vi "Get Data.vi"(8 "error in":errorcluster, 11 "cCRDS in":refnum<class "cCRDS.lvclass">=refnum) -> (0 "error out":errorcluster, 3 "cCRDS_new out":refnum<class "cCRDS.lvclass">)   [LabVIEW 2015, in "cCRDS.lvclass"]
doc: "Retrieve the data from the given cards. All data is acquired in parallel (from the serial ports and the two analog cards). Set the <B>goodData</B> flag to True and log any errors that will be handled down the line. If there is an error associated with the collection of the data, the <B>goodData</B> flag will be set to false when the logged errors are handled.\nThe ringdown traces recorded in the <B>HF AI</B> task are divided up into a m x n matrix where:\n * m = YAG pulse rate\n * n = YAG duty cycle * HF AI Sampling Rate / YAG Pulse Rate\n\nIn the serial data, the first five elements will be the flow controller data. The first element corresponds to the purge flow with the next as follows: thermodenuded (2), dry (4), med RH (1) and high RH (1). \n\nIn the low frequency data, the first twelve elements correpsond to the T, RH and P in the 4 banks of cells. The T and P measured at the output of the banks is assumed to be constant through the banks. The next two signals are the two humidified inputs and the remaining inputs are reserved for thermistor data."
uses:
  cCRDS.lvclass
  Data/cCRDS Data.lvclass
  Reusable/Instrument/state.ctl
  Data/cCRDS Data.lvclass/cCRDS Data.ctl
  Reusable/CRDS/Data/Cell/calData.ctl
  Reusable/CRDS/Cell/CRDS Cell.lvclass/CRDS Cell.ctl
  Reusable/CRDS/Main/Read Cells.vi
  Data Access/Read LF AI.vi
  Data Access/Read SerialIO.vi
  Reusable/CRDS/Data/Main/Write CellData.vi
  Reusable/CRDS/Main/Write Cells.vi
  Reusable/CRDS/Main/Write goodData.vi
  Reusable/CRDS/Cell/CRDS Cell.lvclass
  Reusable/CRDS/Data/Main/CRDS Data.lvclass
  Devices/Alicat/Session Based/Alicat Device.lvclass
  Reusable/CRDS/Data/Cell/CRDS Cell Data.lvclass
  Reusable/Instrument/Instrument.lvclass
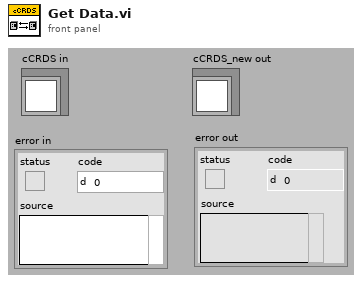
[diagram p1: front panel]
types:
  T1 = typedef "Instrument.lvclass/state.ctl" = enum8{"Configure", "Acquire", "Wait", "Quit", "Handle Error", "NOOP"}
  T2 = typedef "calData.ctl" = cluster{"rhDilFac":sgl, "Q":sgl, "Tmean":sgl, "extDilFac":sgl, "rhCell":sgl, "P":sgl, "T":sgl}
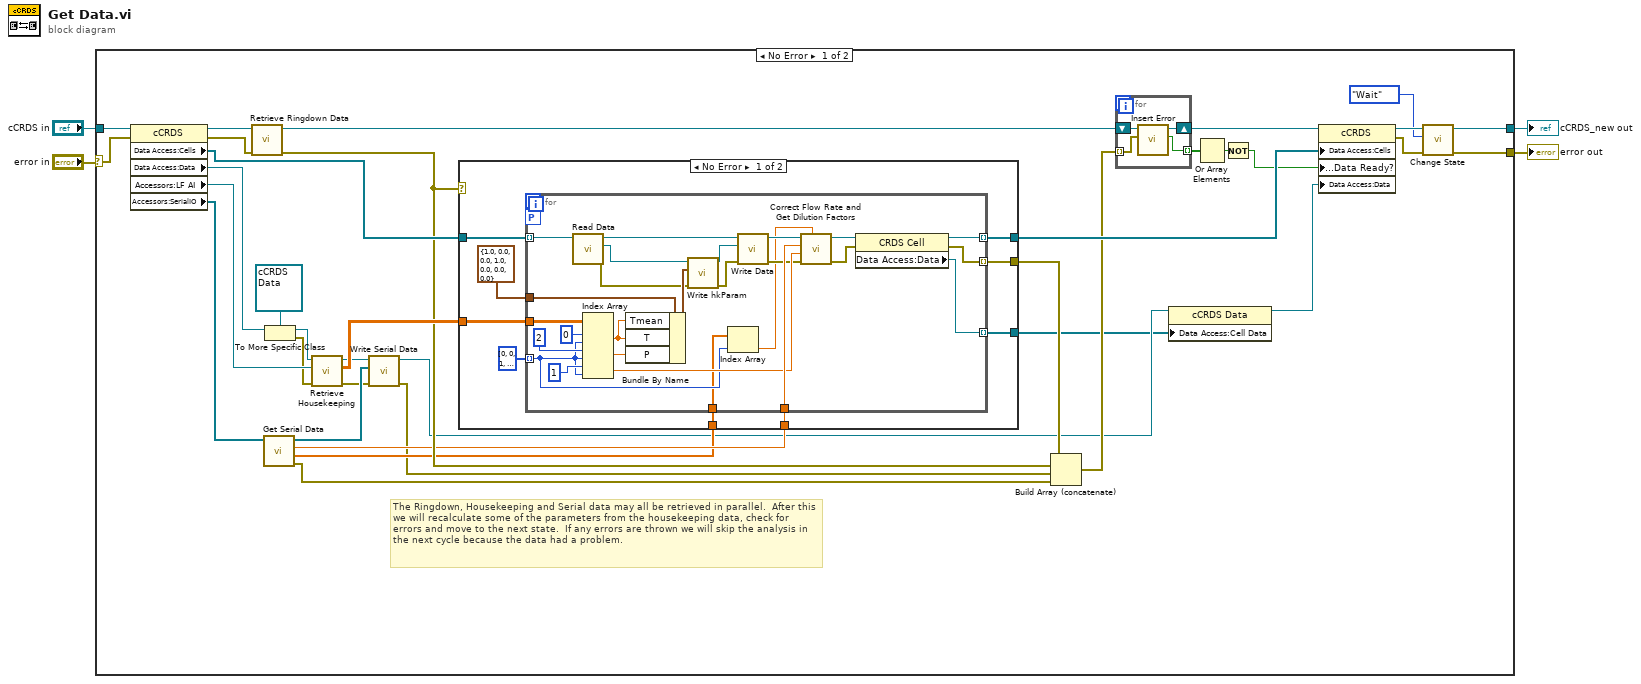
[diagram p0: block diagram]
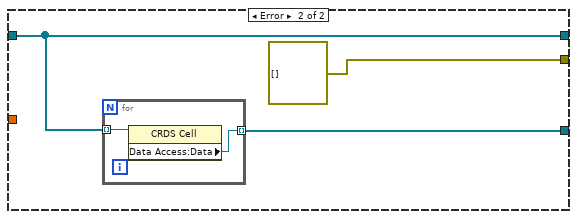
[diagram p2: hidden frame]
diagram:
  n1 = case shown="No Error" "error in" {
    selector: "error in" -> [w39 w86]
    tunnel: [w37 w86] -> w3
    tunnel: "cCRDS in" -> [w40 w85]
    tunnel: [w38 w85] -> w1
    frame No Error {
      # "The Ringdown, Housekeeping and Serial data may all be retrieved in parallel.  After this we will recalculate some of the parameters from the housekeeping data, check for errors and move to the next state.  If any errors are thrown we will skip the analysis in the next cycle because the data had a problem."
      n2 = property class="cCRDS"(reference=w40, error in=w39) -> (reference out=w29:refnum<class "cCRDS.lvclass">, error out=w30:errorcluster, "Data Access:Cells"=w27:refnum<class "CRDS Cell.lvclass">[], "Data Access:Data"=w23:refnum<class "CRDS Data.lvclass">, "Accessors:LF AI"=w26:refnum<k21>, "Accessors:SerialIO"=w12:refnum<class "Alicat Device.lvclass">[])
      n3 = call "Retrieve Ringdown Data.vi"("error in"=w30, "cCRDS in"=w29) -> ("error out"=w20:errorcluster, "cCRDS out"=w28:refnum<class "cCRDS.lvclass">)  [unwired: 8 in]
      n4 = call "Get Serial Data.vi"("SerialIO"=w12) -> ("error out"=w17:errorcluster, "flows"=w18:sgl[], "purge"=w19:sgl, "DataOut"=w10:refnum<class "Data.lvclass">[])  [unwired: 7 in]
      n5 = To More Specific Class(target class=refnum<class "cCRDS Data.lvclass"> refnum ("cCRDS Data"), reference=w23) -> (specific class reference=w25:refnum<class "cCRDS Data.lvclass">, error out=w22:errorcluster)  [unwired: 1 in]
      n6 = call "Retrieve Housekeeping.vi"("error in"=w22, "LF AI"=w26, "CRDS Data In"=w25) -> ("error out"=w9:errorcluster, "Data Out"=w24:sgl[][], "CRDS Data Out"=w11:refnum<class "cCRDS Data.lvclass">)  [unwired: 6 in]
      n7 = call "Write Serial Data.vi"("error in (no error)"=w9, "Serial Data"=w10, "cCRDS Data in"=w11) -> ("error out"=w8:errorcluster, "cCRDS Data out"=w7:refnum<class "cCRDS Data.lvclass">)  [unwired: 7 in]
      n8 = case shown="No Error" w20 {
        tunnel: w27 -> [w53 w81]
        tunnel: [w52 w81] -> w32
        tunnel: [w51 errorcluster[] []] -> w21
        tunnel: w18 -> [w50 _]
        tunnel: w19 -> [w49 _]
        tunnel: w24 -> [w46 _]
        tunnel: [w45 w80] -> w6
        frame No Error {
          n9 = for {
            workers-P: _ -> [_]
            tunnel: w53 -> [w69] mode=indexing
            tunnel: [w55] -> w52 mode=indexing
            tunnel: w50 -> [w60]
            tunnel: w49 -> [w79]
            tunnel: w46 -> [w78]
            tunnel: i32[] [0, 0, 1, 1, 1, 1, 2, 3] -> [w71] mode=indexing
            tunnel: [w56] -> w51 mode=indexing
            tunnel: T2 {"rhDilFac"=1.0, "Q"=0.0, "Tmean"=0.0, "extDilFac"=1.0, "rhCell"=0.0, "P"=0.0, "T"=0.0} ("Housekeeping") -> [w70]
            tunnel: [w54] -> w45 mode=indexing
            n10 = call "Read Data.vi"("CRDS Cell in"=w69) -> ("error out"=w63:errorcluster, "CRDS Cell"=w64:refnum<class "CRDS Cell Data.lvclass">, "CRDS Cell out"=w68:refnum<class "CRDS Cell.lvclass">)  [unwired: 8 in]
            n11 = Index Array(array=w78, index (row) #1=0 ("disabled index (row)"), index (col) #1=w71, index (row) #2=2 ("disabled index (row)"), index (col) #2=w71, index (row) #3=1 ("disabled index (row)"), index (col) #3=w71) -> (element #1=w72:sgl, element #2=w77:sgl, element #3=w73:sgl)
            n12 = Bundle By Name(cluster=w70, "Tmean"=w72, "T"=w72, "P"=w77) -> (w65:T2)
            n13 = call "Write hkParam.vi"("error in (no error)"=w63, "hkParam"=w65, "CRDS Cell Data in"=w64) -> ("error out"=w62:errorcluster, "CRDS Cell Data out"=w66:refnum<class "CRDS Cell Data.lvclass">)  [unwired: 7 in]
            n14 = Index Array(array=w60, index=w71) -> (element=w59:sgl)
            n15 = call "Write Data.vi"("error in"=w62, "CRDS Cell"=w66, "CRDS Cell in"=w68) -> ("error out"=w61:errorcluster, "CRDS Cell out"=w67:refnum<class "CRDS Cell.lvclass">)  [unwired: 7 in]
            n16 = call "Correct Flow Rate and Get Dilution Factors.vi"("Qbank"=w59, "error in"=w61, "RHbank"=w73, "Qpurge"=w79, "CRDS Cell in"=w67) -> ("error out"=w57:errorcluster, "CRDS Cell out"=w58:refnum<class "CRDS Cell.lvclass">)  [unwired: 5 in]
            n17 = property class="CRDS Cell"(reference=w58, error in=w57) -> (reference out=w55:refnum<class "CRDS Cell.lvclass">, error out=w56:errorcluster, "Data Access:Data"=w54:refnum<class "CRDS Cell Data.lvclass">)
          }
        }
        frame Error {
          n18 = for {
            tunnel: w81 -> [w84] mode=indexing
            tunnel: [w83] -> w80 mode=indexing
            n19 = property class="CRDS Cell"(reference=w84) -> ("Data Access:Data"=w83:refnum<class "CRDS Cell Data.lvclass">)  [unwired: 1 in, 2 out]
          }
        }
      }
      n20 = Build Array (concatenate)(w21, w20, w8, w17) -> (w16:errorcluster[])
      n21 = for {
        tunnel: [w43] -> w15 mode=indexing
        shift-right: [w44] -> w31
        shift-left: w28 -> [w42]
        tunnel: w16 -> [w41] mode=indexing
        n22 = call "Insert Error.vi"("err"=w41, "Instrument in"=w42) -> ("error?"=w43:bool, "Instrument out"=w44:refnum<class "cCRDS.lvclass">)  [unwired: 7 in, 1 out]
      }
      n23 = property class="cCRDS Data"(reference=w7, "Data Access:Cell Data"=w6) -> (reference out=w5:refnum<class "cCRDS Data.lvclass">)  [unwired: 1 in, 1 out]
      n24 = Or Array Elements(Boolean array=w15) -> (logical OR=w14:bool)
      n25 = Not(x=w14) -> (.not. x?=w13:bool)
      n26 = property class="cCRDS"(reference=w31, "Data Access:Cells"=w32, "Data Access:Data Ready?"=w13, "Data Access:Data"=w5) -> (reference out=w36:refnum<class "cCRDS.lvclass">, error out=w35:errorcluster)  [unwired: 1 in]
      n27 = call "Change State.vi"("error in"=w35, "instr state"=state."Wait", "Instrument in"=w36) -> ("error out"=w37:errorcluster, "Instrument out"=w38:refnum<class "cCRDS.lvclass">)  [unwired: 7 in]
    }
    frame Error {
    }
  }
  "error out" <- w3
  "cCRDS_new out" <- w1
